vi "Init.vi"(8 "error in (no error)":errorcluster, 10 "Instrument Ref":variant, 11 "Keysight 5700C in":refnum<class "Keysight 5700C.lvclass">) -> (0 "error out":errorcluster, 2 "Found?":bool, 3 "Keysight 5700C out":refnum<class "Keysight 5700C.lvclass">)   [LabVIEW 2025, in "Power Supply.lvlib" / "Keysight 5700C.lvclass"]
uses:
  Keysight 5700C.lvclass
  Keysight 5700C.lvclass/Keysight 5700C.ctl
  Users/Public/Documents/Sandia National Labs/TSS Plugin/Abstract Engine.lvlibp/Instrument configuration/Instrument configuration.lvclass
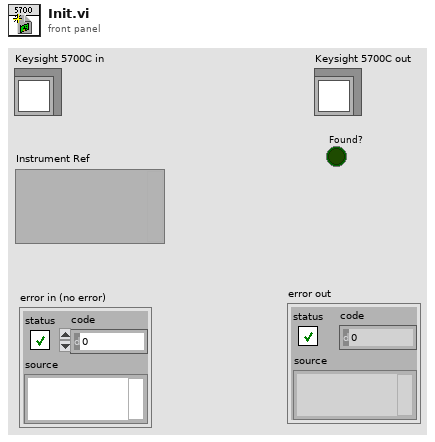
[diagram p1: front panel]
types:
  T1 = typedef "Abstract Engine.lvlibp/Instrument configuration.lvclass/Default Instrument.ctl" = cluster{"Type":string, "Address":string, "SW Alias":string, "Description":string, "Enabled":bool}
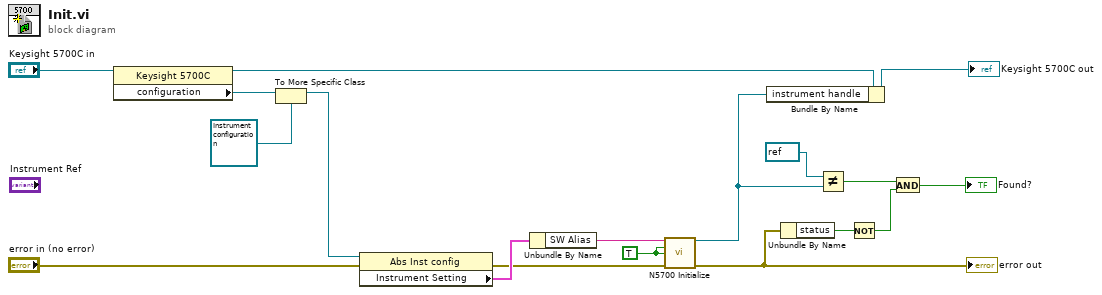
[diagram p0: block diagram]
diagram:
  w5 = TRUE ("id query (Yes)")
  n1 = property class="Keysight 5700C"(reference="Keysight 5700C in") -> (reference out=w14:refnum<class "Keysight 5700C.lvclass">, "configuration"=w16:refnum<class "CEF_serializable configuration.lvclass">)  [unwired: 1 in, 1 out]
  n2 = To More Specific Class(target class=refnum<class "Instrument configuration.lvclass"> refnum ("Abstract PlugIn.lvlibp:Instrument configuration"), reference=w16) -> (specific class reference=w17:refnum<class "Instrument configuration.lvclass">)  [unwired: 1 in, 1 out]
  n3 = property class="Abs Inst config"(reference=w17, error in="error in (no error)") -> (error out=w4:errorcluster, "Instrument Setting"=w6:T1)  [unwired: 1 out]
  n4 = Unbundle By Name(w6) -> ("SW Alias"=w2:string)
  n5 = call <instrlib>:"N5700 Initialize.vi"("VISA name"=w2, "ID Query (T)"=w5, "Reset (T)"=w5, "error in (no error)"=w4) -> ("VISA out"=w1:refnum<visa-resource-name>, "error out"=w3:errorcluster)  [unwired: 10 in]
  "error out" <- w3
  n6 = Bundle By Name(cluster=w14, "instrument handle"=w1) -> (→"Keysight 5700C out":refnum<class "Keysight 5700C.lvclass">)
  n7 = Unbundle By Name(w3) -> ("status"=w11:bool)
  n8 = Not Equal?(x=refnum<visa-resource-name> refnum ("VISA resource name out"), y=w1) -> (x != y?=w10:bool)
  n9 = Not(x=w11) -> (.not. x?=w9:bool)
  n10 = And(x=w10, y=w9) -> (x .and. y?=→"Found?":bool)
